vi "polar_to_cartesian.vi"(2 "B (T)":dbl min=0.0 format="%.3f", 3 "Phi (Deg)":dbl format="%#_13g") -> (0 "Z Field (T)":dbl format="%#_13g", 1 "Y Field (T)":dbl format="%#_13g")   [LabVIEW 2019]
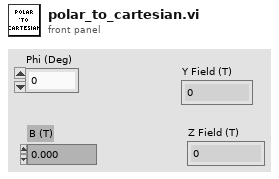
[diagram p1: front panel]
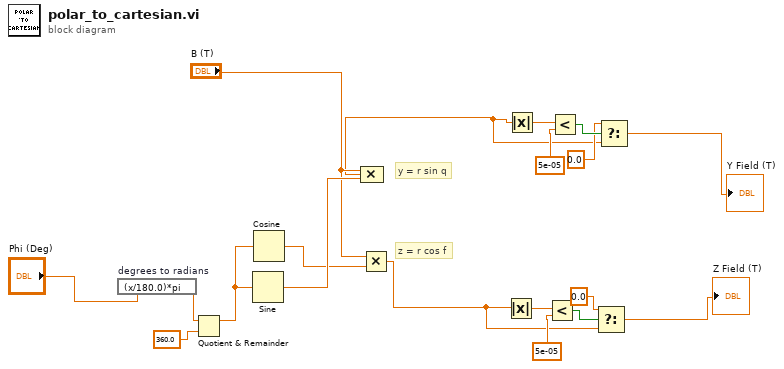
[diagram p0: block diagram]
diagram:
  # "z = r cos f"
  # "y = r sin q"
  n1 = expression code="(x/180.0)*pi" "degrees to radians"("Phi (Deg)") -> (w15:dbl)
  n2 = Quotient & Remainder(x=w15, y=360.0) -> (x-y*floor(x/y)=w13:dbl)  [unwired: 1 out]
  n3 = Sine(x=w13) -> (sin(x)=w19:dbl)
  n4 = Cosine(x=w13) -> (cos(x)=w18:dbl)
  n5 = Compound Arithmetic op=MULTIPLY("B (T)", w19) -> (w4:dbl)
  n6 = Multiply(x="B (T)", y=w18) -> (x*y=w2:dbl)
  n7 = Absolute Value(x=w2) -> (abs(x)=w1:dbl)
  n8 = Absolute Value(x=w4) -> (abs(x)=w3:dbl)
  n9 = Less?(x=w1, y=5e-05) -> (x < y?=w10:bool)
  n10 = Less?(x=w3, y=5e-05) -> (x < y?=w12:bool)
  n11 = Select(t=0.0, s=w10, f=w2) -> (s? t:f=→"Z Field (T)":dbl)
  n12 = Select(t=0.0, s=w12, f=w4) -> (s? t:f=→"Y Field (T)":dbl)
